vi "Minimo.vi"(8 "error in (no error)":errorcluster, 10 "Minimo":u8, 11 "Measurement_Binary in":refnum<class "Measurement_Binary.lvclass">) -> (0 "error out":errorcluster, 3 "Measurement_Binary out":refnum<class "Measurement_Binary.lvclass">)   [LabVIEW 2020, in "Measurement_Binary.lvlib" / "Measurement_Binary.lvclass"]
uses:
  Measurement_Binary.lvclass
  Measurement_Binary.lvclass/Measurement_Binary.ctl
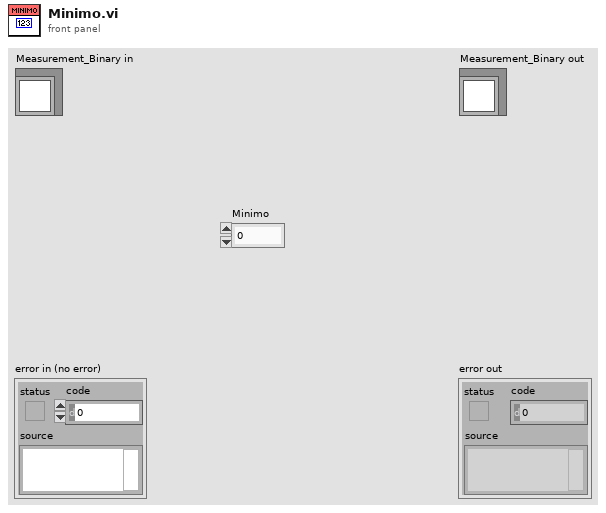
[diagram p1: front panel]
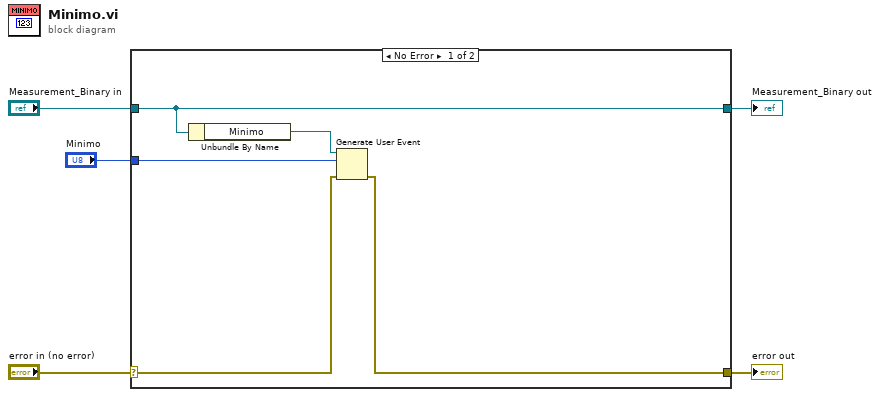
[diagram p0: block diagram]
diagram:
  n1 = case shown="No Error" "error in (no error)" {
    selector: "error in (no error)" -> [w7 w12]
    tunnel: [w6 w12] -> w4
    tunnel: [w10 w11] -> w2
    tunnel: "Measurement_Binary in" -> [w10 w11]
    tunnel: "Minimo" -> [w8 _]
    frame No Error {
      n2 = Unbundle By Name(w10) -> ("Minimo"=w9:refnum<user-event>)
      n3 = Generate User Event(user event=w9, event data cluster=w8, error in=w7) -> (error out=w6:errorcluster)  [unwired: 1 in, 1 out]
    }
    frame Error {
    }
  }
  "error out" <- w4
  "Measurement_Binary out" <- w2
